vi "Teleop.vi"(10 "Match Info":T1={"Autonomous Elapsed Seconds"=0.0, "TeleOp Elapsed Seconds"=0.0, "Disabled Elapsed Seconds"=0.0, "Visited Autonomous"=FALSE, "Visited TeleOp"=FALSE, "Visited Disabled"=FALSE, "Autonomous Settings"={"Autonomous Style"=enum."Independent", "VI Refnum"=refnum}}, 11 "Call Context":T2) -> ()   [LabVIEW 2016]
doc: "This VI is called for each TeleOp packet received from the DS where the robot is not disabled. It is often used to read from the joysticks and update I/O or to update setpoints for timed control loops. It should complete and return within 20 milliseconds or it may miss DS packets."
uses:
  <vilib>/Rock Robotics/WPI/DriverStation/WPI_DriverStationDerivedRobotMode.ctl
  <vilib>/Rock Robotics/WPI/DriverStation/WPI_DriverStationMatch Info.ctl
  <vilib>/Rock Robotics/WPI/ThirdParty/CanMotor/TalonSRX/WPI_CANTalonSRX_APIFeedbackSelect.ctl
  <vilib>/Rock Robotics/WPI/ThirdParty/CanMotor/TalonSRX/WPI_CANTalonSRX_APIControlMode.ctl
  <vilib>/Rock Robotics/WPI/Utilities/WPI_GetSetVariantRefNum.vi
  <vilib>/Rock Robotics/Network Tables/NT Write Boolean Array.vi
  <vilib>/Rock Robotics/Network Tables/NT Write Numeric Array.vi
  <vilib>/Rock Robotics/Network Tables/NT Read Boolean.vi
  <vilib>/Rock Robotics/Network Tables/NT Read Number.vi
  Robot Global Data.vi
  <vilib>/Rock Robotics/Network Tables/NT Write Boolean.vi
panel:
  out "Value 2":bool
  out "Value":bool
  out "Left Encoder":dbl
  out "Right Encoder":dbl
  out "Battery Voltage":dbl
  out "Current":dbl
  out "SensorPosRotations":dbl
  out "Motor output Plot":cluster{"Applied Throttle":dbl}(graph)
  out "Target RPM":dbl
  out "SensorRPM Velocity RPM":dbl
  out "Applied Output":dbl
  out "Speed Closed Loop Plots":cluster{dbl, "Sensor Velocity":dbl}(graph)
  in  "Enable":bool=TRUE
  in  "Reset":bool
  out "Table":string[][](table)
  out "Encoder Velocity":dbl
  out "Sample Slider 0":dbl(slide) scale=0.0..5.0
  out "Sample Boolean 1":bool
  out "Sample Boolean 0":bool
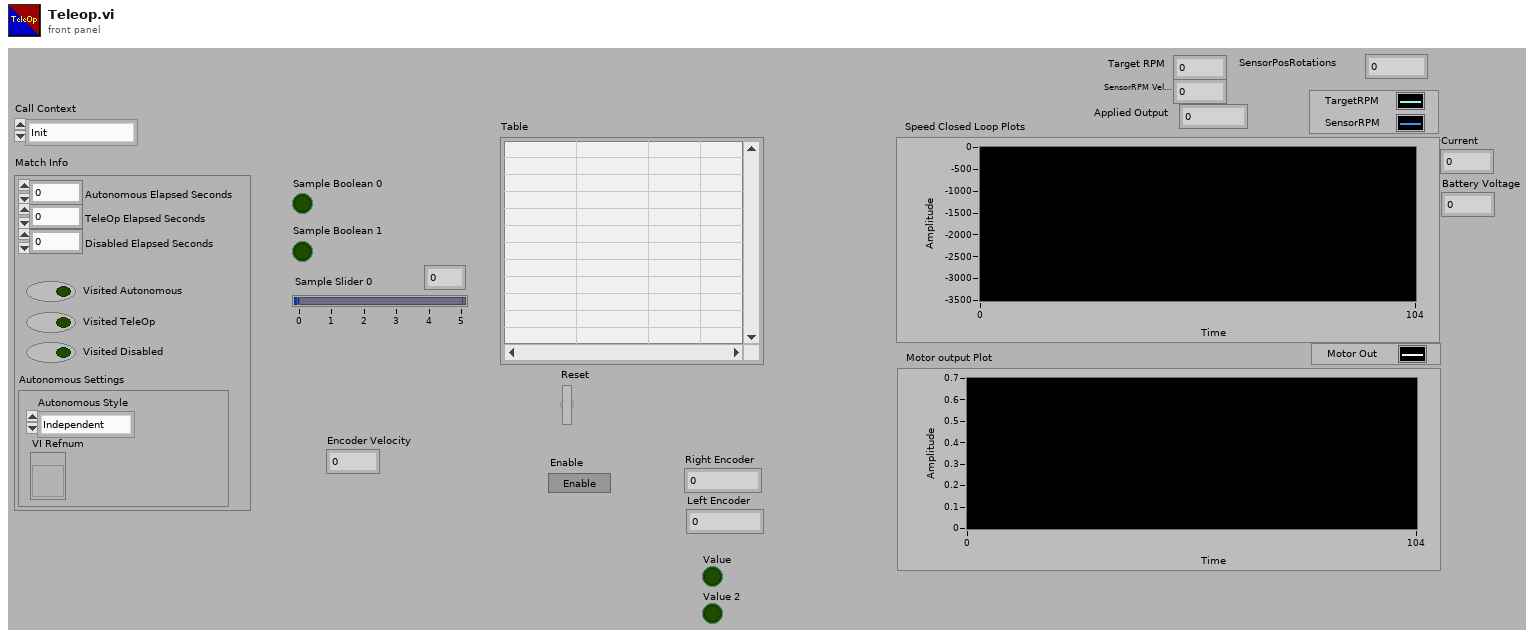
[diagram p1: front panel]
types:
  T1 = typedef "WPI_DriverStationMatch Info.ctl" = cluster{"Autonomous Elapsed Seconds":dbl, "TeleOp Elapsed Seconds":dbl, "Disabled Elapsed Seconds":dbl, "Visited Autonomous":bool, "Visited TeleOp":bool, "Visited Disabled":bool, "Autonomous Settings":cluster{"Autonomous Style":enum16{"Iterative", "Independent"}, "VI Refnum":refnum<vi>}}
  T2 = typedef "WPI_DriverStationDerivedRobotMode.ctl" = enum16{"Init", "Execute", "Stop"}
  T3 = typedef "WPI_CANTalonSRX_APIFeedbackSelect.ctl" = enum16{"Digital Quadrature Encoder", "Analog Potentiometer", "Analog Encoder", "Count on Quad-A (Rising-Edge)", "Count on Quad-A (Falling-Edge)", "CTR Magnetic Enc (Absolute)", "CTR Magnetic Enc (Relative)", "Pulse Width"}
  T4 = typedef "WPI_JoystickDevRef.ctl" = cluster{"Device":T5}
  T5 = typedef "WPI_JoystickDeviceEnum.ctl" = enum16{"USB 0", "USB 1", "USB 2", "USB 3", "USB 4", "USB 5"}
  T6 = typedef "WPI_RobotDriveDevRef.ctl" = cluster{"DevStatus":errorcluster, "Motors[]":T7[], "Square Inputs":bool, "Max Output":dbl}
  T7 = typedef "WPI_MotorControlDeviceRef.ctl" = cluster{"DeviceStatus":errorcluster, "Type":T8, "PWM":cluster{"PWM Channel":T9, "DeadBand":T10}, "CAN":cluster{"Device Number":u8, "SetOutput VI Ref":variant, "GetOutput VI Ref":variant, "Enable VI Ref":variant, "Disable VI Ref":variant, "Data":variant}, "Invert":bool}
  T8 = typedef "WPI_MotorControlType.ctl" = enum16{"PWM", "CAN"}
  T9 = typedef "FPGA_DIOPWMChannel.ctl" = enum8{"PWM 0", "PWM 1", "PWM 2", "PWM 3", "PWM 4", "PWM 5", "PWM 6", "PWM 7", "PWM 8", "PWM 9", "PWM MXP 0", "PWM MXP 1", "PWM MXP 2", "PWM MXP 3", "PWM MXP 4", "PWM MXP 5", "PWM MXP 6", "PWM MXP 7", "PWM MXP 8", "PWM MXP 9", "Invalid"}
  T10 = typedef "WPI_PWMDeadband.ctl" = cluster{"Name":string, "maxPositivePwm":i32, "minPositivePwm":i32, "centerPwm":i32, "maxNegativePwm":i32, "minNegativePwm":i32, "angularRange":u16}
  T11 = typedef "WPI_EncoderDevRef.ctl" = cluster{"DevStatus":errorcluster, "EncoderIndex":T12, "CounterIndex":T13, "DistancePerCount":dbl, "Decoding Type":T14}
  T12 = typedef "FPGA_EncoderIdx.ctl" = enum8{"Enc 0", "Enc 1", "Enc 2", "Enc 3", "Enc 4", "Enc 5", "Enc 6", "Enc 7", "Invalid"}
  T13 = typedef "FPGA_CounterCtrSystemIndex.ctl" = enum8{"Ctr 0", "Ctr 1", "Ctr 2", "Ctr 3", "Ctr 4", "Ctr 5", "Ctr 6", "Ctr 7", "Invalid"}
  T14 = typedef "WPI_EncoderType.ctl" = enum16{"1x", "2x", "4x"}
  T15 = typedef "WPI_CANTalonSRX_GlobalStatus.ctl" = cluster{"Applied Throttle":dbl, "Module Enabled":bool, "CAN Error":errorcluster, "Closed Loop Error":dbl, "Forward Limit Switch Closed":bool, "Reverse Limit Switch Closed":bool, "Sensor Position":dbl, "Sensor Velocity":dbl, "Current":dbl, "Sticky Fault - Over Temp":bool, "Sticky Fault - Under Voltage":bool, "Sticky Fault - Forward Limit":bool, "Sticky Fault - Reverse Limit":bool, "Sticky Fault - Forward Soft Limit":bool, "Sticky Fault - Reverse Soft Limit":bool, "Brake is Enabled":bool, "Encoder Position":dbl, "Encoder Velocity":dbl, "Encoder Index Count":dbl, "Encoder A Pin State":bool, "Encoder B Pin State":bool, "Encoder Index Pin State":bool, "Analog In":dbl, "Analog In Velocity":dbl, "Temperature (C)":dbl, "Battery Voltage":dbl, "Control 5 Is Supported":bool, "Current Profile Slot Select":dbl, "Pos Div 8":bool, "Vel Div 4":bool, "Pulse Width Position":i32, "Pulse Width Velocity":i32, "Pulse Width Rise To Rise (us)":i32, "Pulse Width Rise To Fall (us)":i32, "Mot Prof Active Is Under Run":bool, "Mot Prof Active Has Under Run":bool, "Mot Prof Active Is Last":bool, "Mot Prof Active Velocity Only":bool, "Mot Prof Active Is Valid":bool, "Mot Prof Buffer Is Full":bool, "Mot Prof Active Profile Slot Select":i32, "Mot Prof NextID":i32, "Mot Prof Count":i32, "Mot Prof Active Velocity":dbl, "Mot Prof Active Position":dbl, "Mot Prof Output Enable":i32, "UsageFrame":u32}
  T16 = typedef "WPI_DigitalInputDevRef.ctl" = cluster{"DevStatus":errorcluster, "DIO Channel":T17}
  T17 = typedef "FPGA_DIOChannel.ctl" = enum8{"DIO 0", "DIO 1", "DIO 2", "DIO 3", "DIO 4", "DIO 5", "DIO 6", "DIO 7", "DIO 8", "DIO 9", "DIO MXP 0", "DIO MXP 1", "DIO MXP 2", "DIO MXP 3", "DIO MXP 4", "DIO MXP 5", "DIO MXP 6", "DIO MXP 7", "DIO MXP 8", "DIO MXP 9", "DIO MXP 10", "DIO MXP 11", "DIO MXP 12", "DIO MXP 13", "DIO MXP 14", "DIO MXP 15", "SPI Port CS1", "SPI Port CS2", "SPI Port CS3", "SPI Port MISO", "SPI Port MOSI", "Invalid"}
  T18 = typedef "WPI_CANTalonSRX_APIControlMode.ctl" = enum8{"Percent VBus", "Speed", "Position", "Slave", "Unchanged / Invalid", "Voltage Compensation", "Current", "Motion Profile", "Motion Magic"}
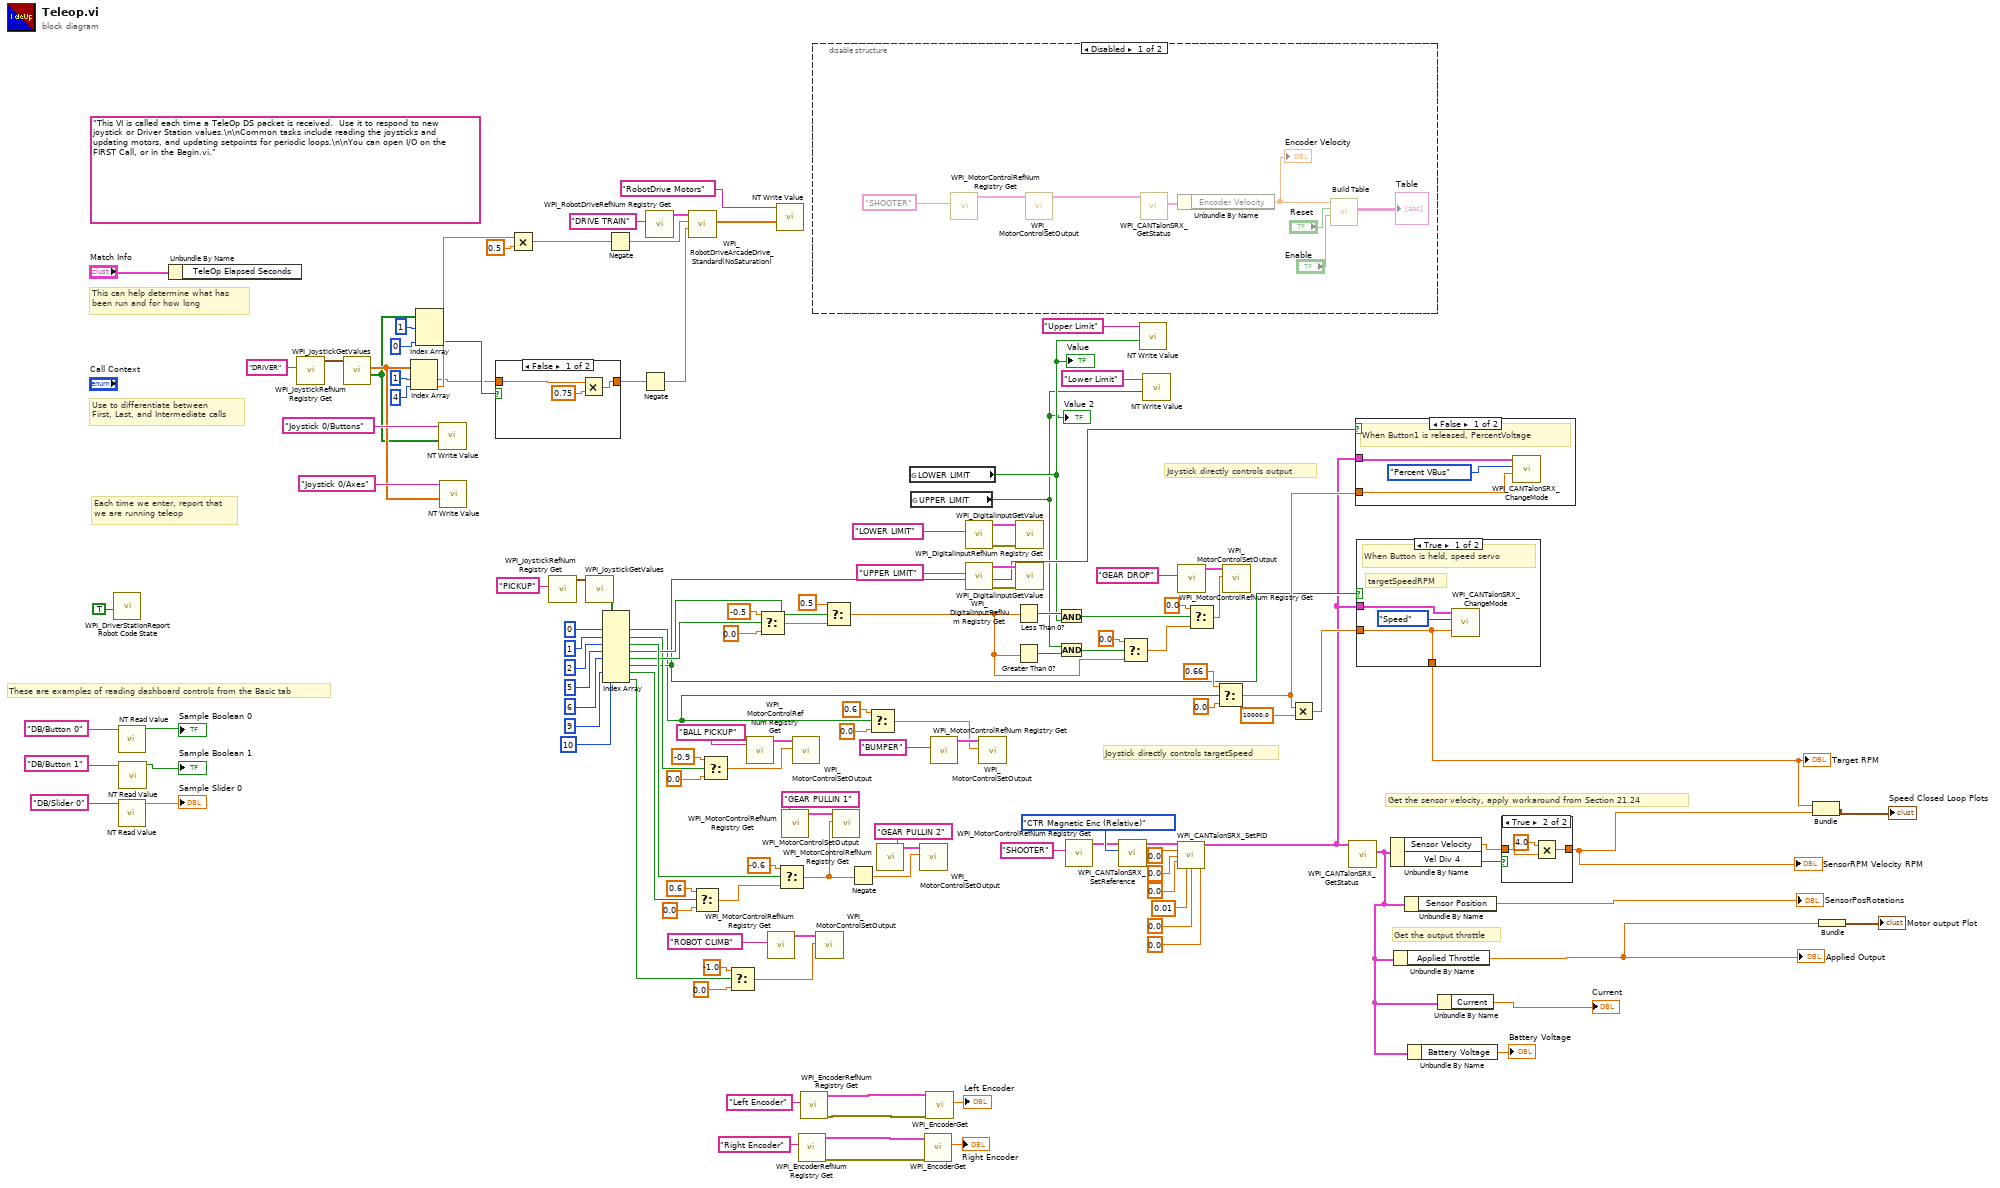
[diagram p0: block diagram]
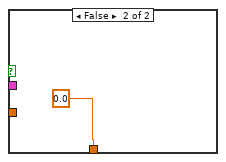
[diagram p6: hidden frame]
diagram:
  (unwired) "This VI is called each time a TeleOp DS packet is received.  Use it to respond to new joystick or Driver Station values.\n\nCommon tasks include reading the joysticks and updating motors, and updating setpoints for periodic loops.\n\nYou can open I/O on the FIRST Call, or in the Begin.vi."
  # "Get the output throttle"
  # "Get the sensor velocity, apply workaround from Section 21.24"
  # "Joystick directly controls targetSpeed"
  # "Joystick directly controls output"
  # "These are examples of reading dashboard controls from the Basic tab"
  # "Each time we enter, report that\nwe are running teleop"
  # "Use to differentiate between\nFirst, Last, and Intermediate calls"
  # "This can help determine what has\nbeen run and for how long"
  n1 = call <vilib>:"WPI_DriverStationReport Robot Code State.vi"("TeleOp"=TRUE ("Autonomous")) -> ()  [unwired: 10 in, 1 out]
  n2 = call-poly <vilib>:"NT Read Value.vi"("Name"="DB/Button 0" ("refnum name")) -> ("Boolean"=→"Sample Boolean 0":bool)  [unwired: 9 in, 1 out]
  n3 = call-poly <vilib>:"NT Read Value.vi"("Name"="DB/Slider 0" ("refnum name")) -> ("Numeric"=→"Sample Slider 0":dbl)  [unwired: 9 in, 1 out]
  n4 = call-poly <vilib>:"NT Read Value.vi"("Name"="DB/Button 1" ("refnum name")) -> ("Boolean"=→"Sample Boolean 1":bool)  [unwired: 9 in, 1 out]
  n5 = Unbundle By Name("Match Info") -> ()  [unwired: 1 out]
  n6 = call <vilib>:"WPI_JoystickRefNum Registry Get.vi"("refnum name"="DRIVER") -> ("JoystickDevRef"=w129:T4)  [unwired: 1 in, 9 out]
  n7 = call <vilib>:"WPI_JoystickGetValues.vi"("JoystickDevRef"=w129) -> ("Buttons"=w87:bool[], "Axes"=w125:dbl[])  [unwired: 6 in, 3 out]
  n8 = Index Array(array=w125, index #1=1 ("index"), index #2=4 ("index")) -> (element #1=w30:dbl, element #2=w83:dbl)
  n9 = Index Array(array=w87, index #1=1 ("index"), index #3=0 ("index")) -> (element #3=w31:bool)  [unwired: 1 in, 2 out]
  n10 = call-poly <vilib>:"NT Write Value.vi"("Boolean Array"=w87, "Name"="Joystick 0/Buttons") -> ()  [unwired: 9 in, 1 out]
  n11 = call-poly <vilib>:"NT Write Value.vi"("Numeric Array"=w125, "Name"="Joystick 0/Axes") -> ()  [unwired: 9 in, 1 out]
  n12 = case shown="False" w31 {
    tunnel: [w135 w137] -> w29
    tunnel: w30 -> [w134 w137]
    frame False {
      n13 = Multiply(x=w134, y=0.75) -> (x*y=w135:dbl)
    }
    frame True {
    }
  }
  n14 = Multiply(x=w83, y=0.5) -> (x*y=w74:dbl)
  n15 = call <vilib>:"WPI_JoystickRefNum Registry Get.vi"("refnum name"="PICKUP") -> ("JoystickDevRef"=w116:T4)  [unwired: 1 in, 9 out]
  n16 = call <vilib>:"WPI_JoystickGetValues.vi"("JoystickDevRef"=w116) -> ("Buttons"=w114:bool[])  [unwired: 6 in, 4 out]
  n17 = Index Array(array=w114, index #1=0 ("index"), index #2=1 ("index"), index #3=2 ("index"), index #4=5 ("index"), index #5=6 ("index"), index #7=9 ("index"), index #8=10 ("index")) -> (element #1=w39:bool, element #2=w90:bool, element #3=w97:bool, element #4=w96:bool, element #5=w95:bool, element #6=w42:bool, element #7=w25:bool, element #8=w13:bool)  [unwired: 1 in]
  n18 = Negate(x=w74) -> (-x=w73:dbl)
  n19 = Negate(x=w29) -> (-x=w75:dbl)
  n20 = call <vilib>:"WPI_RobotDriveRefNum Registry Get.vi"("refnum name"="DRIVE TRAIN") -> ("RobotDriveDevRef"=w131:T6)  [unwired: 1 in, 9 out]
  n21 = call <vilib>:"WPI_RobotDriveArcadeDrive_Standard(NoSaturation).vi"("Y axis value"=w75, "X axis value"=w73, "RobotDriveDevRef"=w131) -> ("Motor Values"=w118:dbl[])  [unwired: 1 in, 7 out]
  n22 = Select(t=0.6, s=w25, f=0.0) -> (s? t:f=w27:dbl)
  n23 = Select(t=-0.9, s=w90, f=0.0) -> (s? t:f=w92:dbl)
  n24 = Select(t=-1.0, s=w13, f=0.0) -> (s? t:f=w16:dbl)
  n25 = call <vilib>:"WPI_MotorControlRefNum Registry Get.vi"("refnum name"="BALL PICKUP") -> ("MotorControlDevRef"=w94:T7)  [unwired: 9 in, 1 out]
  n26 = Select(t=-0.5, s=w95, f=0.0) -> (s? t:f=w71:dbl)
  n27 = call <vilib>:"WPI_MotorControlRefNum Registry Get.vi"("refnum name"="ROBOT CLIMB") -> ("MotorControlDevRef"=w17:T7)  [unwired: 9 in, 1 out]
  n28 = call-poly <vilib>:"NT Write Value.vi"("Numeric Array"=w118, "Name"="RobotDrive Motors") -> ()  [unwired: 9 in, 1 out]
  n29 = Select(t=-0.6, s=w97, f=w27) -> (s? t:f=w107:dbl)
  n30 = call <vilib>:"WPI_MotorControlRefNum Registry Get.vi"("refnum name"="GEAR PULLIN 1") -> ("MotorControlDevRef"=w112:T7)  [unwired: 9 in, 1 out]
  n31 = call <vilib>:"WPI_MotorControlSetOutput.vi"("Output"=w92, "MotorControlDevRef"=w94) -> ()  [unwired: 7 in, 3 out]
  n32 = call <vilib>:"WPI_EncoderRefNum Registry Get.vi"("refnum name"="Right Encoder") -> ("error out"=w3:errorcluster, "EncoderDevRef"=w4:T11)  [unwired: 9 in]
  n33 = call <vilib>:"WPI_EncoderRefNum Registry Get.vi"("refnum name"="Left Encoder") -> ("error out"=w5:errorcluster, "EncoderDevRef"=w6:T11)  [unwired: 9 in]
  n34 = disable-structure shown="Disabled" {
    frame Disabled {
      n35 = call <vilib>:"WPI_MotorControlRefNum Registry Get.vi"("refnum name"="SHOOTER") -> ("MotorControlDevRef"=w138:T7)  [unwired: 9 in, 1 out]
      n36 = call <vilib>:"WPI_MotorControlSetOutput.vi"("MotorControlDevRef"=w138) -> ("MotorControlDevRef"=w145:T7)  [unwired: 8 in, 2 out]
      n37 = call <vilib>:"WPI_CANTalonSRX_GetStatus.vi"("CAN Talon SRX Ref"=w145) -> ("Talon SRX Status"=w144:T15)  [unwired: 8 in, 2 out]
      n38 = Unbundle By Name(w144) -> ("Encoder Velocity"=w142:dbl)
      "Encoder Velocity" <- w142
      n39 = call "Build Table"("Enable"="Enable", "Reset"="Reset", "Signals"=w142) -> ("Table"=→"Table":string[][])  [unwired: 2 in, 6 out]
    }
    frame Enabled {
    }
  }
  n40 = call <vilib>:"WPI_MotorControlSetOutput.vi"("Output"=w16, "MotorControlDevRef"=w17) -> ()  [unwired: 7 in, 3 out]
  n41 = Select(t=0.5, s=w96, f=w71) -> (s? t:f=w65:dbl)
  n42 = call <vilib>:"WPI_MotorControlSetOutput.vi"("Output"=w107, "MotorControlDevRef"=w112) -> ()  [unwired: 7 in, 3 out]
  n43 = Negate(x=w107) -> (-x=w106:dbl)
  n44 = Select(t=0.6, s=w39, f=0.0) -> (s? t:f=w36:dbl)
  n45 = call <vilib>:"WPI_MotorControlRefNum Registry Get.vi"("refnum name"="GEAR PULLIN 2") -> ("MotorControlDevRef"=w109:T7)  [unwired: 9 in, 1 out]
  n46 = global read "Robot Global Data.vi" "LOWER LIMIT"() -> (w2:bool)
  "Value" <- w2
  n47 = global read "Robot Global Data.vi" "UPPER LIMIT"() -> (w1:bool)
  "Value 2" <- w1
  n48 = call <vilib>:"WPI_MotorControlSetOutput.vi"("Output"=w106, "MotorControlDevRef"=w109) -> ()  [unwired: 7 in, 3 out]
  n49 = call <vilib>:"WPI_EncoderGet.vi"("error in (no error)"=w3, "EncoderDevRef"=w4) -> ("Distance"=→"Right Encoder":dbl)  [unwired: 4 in, 5 out]
  n50 = call <vilib>:"WPI_EncoderGet.vi"("error in (no error)"=w5, "EncoderDevRef"=w6) -> ("Distance"=→"Left Encoder":dbl)  [unwired: 4 in, 5 out]
  n51 = call <vilib>:"WPI_MotorControlRefNum Registry Get.vi"("refnum name"="BUMPER") -> ("MotorControlDevRef"=w41:T7)  [unwired: 9 in, 1 out]
  n52 = call <vilib>:"WPI_DigitalInputRefNum Registry Get.vi"("refnum name"="LOWER LIMIT") -> ("error out"=w78:errorcluster, "DigitalInputDevRef"=w79:T16)  [unwired: 9 in]
  n53 = call <vilib>:"WPI_DigitalInputRefNum Registry Get.vi"("refnum name"="UPPER LIMIT") -> ("error out"=w81:errorcluster, "DigitalInputDevRef"=w80:T16)  [unwired: 9 in]
  n54 = call <vilib>:"WPI_MotorControlSetOutput.vi"("Output"=w36, "MotorControlDevRef"=w41) -> ()  [unwired: 7 in, 3 out]
  n55 = Less Than 0?(x=w65) -> (x < 0?=w67:bool)
  n56 = Greater Than 0?(x=w65) -> (x > 0?=w68:bool)
  n57 = call <vilib>:"WPI_DigitalInputGetValue.vi"("error in (no error)"=w78, "DigitalInputDevRef"=w79) -> ()  [unwired: 7 in, 3 out]
  n58 = call <vilib>:"WPI_DigitalInputGetValue.vi"("error in (no error)"=w81, "DigitalInputDevRef"=w80) -> ()  [unwired: 7 in, 3 out]
  n59 = And(x=w67, y=w2) -> (x .and. y?=w69:bool)
  n60 = And(x=w1, y=w68) -> (x .and. y?=w70:bool)
  n61 = call <vilib>:"WPI_MotorControlRefNum Registry Get.vi"("refnum name"="SHOOTER") -> ("MotorControlDevRef"=w53:T7)  [unwired: 9 in, 1 out]
  n62 = call <vilib>:"WPI_CANTalonSRX_SetReference.vi"("Feedback Reference"=WPI_CANTalonSRX_APIFeedbackSelect."CTR Magnetic Enc (Relative)", "CAN Talon SRX Ref"=w53) -> ("CAN Talon SRX Ref"=w52:T7)  [unwired: 8 in, 1 out]
  n63 = Select(t=0.0, s=w70, f=w65) -> (s? t:f=w63:dbl)
  n64 = call-poly <vilib>:"NT Write Value.vi"("Boolean"=w2, "Name"="Upper Limit") -> ()  [unwired: 9 in, 1 out]
  n65 = call-poly <vilib>:"NT Write Value.vi"("Boolean"=w1, "Name"="Lower Limit") -> ()  [unwired: 9 in, 1 out]
  n66 = call <vilib>:"WPI_CANTalonSRX_SetPID.vi"("CAN Talon SRX Ref"=w52, "P"=0.0, "I"=0.0, "D"=0.0, "F"=0.01, "I Zone"=0.0, "Ramp Rate"=0.0) -> ("CAN Talon SRX Ref"=w23:T7)  [unwired: 7 in, 1 out]
  n67 = call <vilib>:"WPI_MotorControlRefNum Registry Get.vi"("refnum name"="GEAR DROP") -> ("MotorControlDevRef"=w104:T7)  [unwired: 9 in, 1 out]
  n68 = Select(t=0.0, s=w69, f=w63) -> (s? t:f=w72:dbl)
  n69 = Select(t=0.66 ("Output"), s=w39, f=0.0) -> (s? t:f=w44:dbl)
  n70 = call <vilib>:"WPI_MotorControlSetOutput.vi"("Output"=w72, "MotorControlDevRef"=w104) -> ()  [unwired: 7 in, 3 out]
  n71 = Multiply(x=w44, y=10000.0) -> (x*y=w47:dbl)
  n72 = call <vilib>:"WPI_CANTalonSRX_GetStatus.vi"("CAN Talon SRX Ref"=w23) -> ("Talon SRX Status"=w34:T15)  [unwired: 8 in, 2 out]
  n73 = case shown="False" w42 {
    tunnel: w23 -> [w147 _]
    tunnel: w44 -> [w146 _]
    frame False {
      # "When Button1 is released, PercentVoltage"
      n74 = call <vilib>:"WPI_CANTalonSRX_ChangeMode.vi"("Output"=w146, "Control Mode"=WPI_CANTalonSRX_APIControlMode."Percent VBus", "CAN Talon SRX Ref"=w147) -> ()  [unwired: 7 in, 2 out]
    }
    frame True {
    }
  }
  n75 = case shown="True" w42 {
    tunnel: w47 -> [w149 _]
    tunnel: w23 -> [w150 _]
    tunnel: [w149 0.0 ("x")] -> w46
    frame True {
      # "targetSpeedRPM"
      # "When Button is held, speed servo"
      n76 = call <vilib>:"WPI_CANTalonSRX_ChangeMode.vi"("Output"=w149, "Control Mode"=WPI_CANTalonSRX_APIControlMode."Speed", "CAN Talon SRX Ref"=w150) -> ()  [unwired: 7 in, 2 out]
    }
    frame False {
    }
  }
  "Target RPM" <- w46
  n77 = Unbundle By Name(w34) -> ("Sensor Velocity"=w56:dbl, "Vel Div 4"=w55:bool)
  n78 = Unbundle By Name(w34) -> ("Applied Throttle"=w48:dbl)
  "Applied Output" <- w48
  n79 = Unbundle By Name(w34) -> ("Sensor Position"=→"SensorPosRotations":dbl)
  n80 = Unbundle By Name(w34) -> ("Battery Voltage"=→"Battery Voltage":dbl)
  n81 = Unbundle By Name(w34) -> ("Current"=→"Current":dbl)
  n82 = case shown="True" w55 {
    tunnel: [w153 w155] -> w54
    tunnel: w56 -> [w153 w154]
    frame False {
    }
    frame True {
      n83 = Multiply(x=4.0, y=w154) -> (x*y=w155:dbl)
    }
  }
  "SensorRPM Velocity RPM" <- w54
  n84 = Bundle("x"=w46, "Sensor Velocity"=w54) -> (→"Speed Closed Loop Plots":cluster{"x":dbl, "Sensor Velocity":dbl})  [unwired: 1 in]
  n85 = Bundle("Applied Throttle"=w48) -> (→"Motor output Plot":cluster{"Applied Throttle":dbl})  [unwired: 1 in]
